vi "Stop Core.vi"(10 "final error code":i32, 11 "Acquisition in":refnum<class "Acquisition.lvclass">) -> (3 "Acquisition out":refnum<class "Acquisition.lvclass">)   [LabVIEW 2018, in "Acquisition.lvlib" / "Acquisition.lvclass"]
doc: "(<B>Filename</B>: Actor Framework.lvlib:Actor.lvclass:Stop Core.vi)\n\nDefines what the actor does before it stops. Use the <B>final error code</B> input to determine whether the actor shut down in response to an error.\n\nBy default, this method passes the Stop message along to all auto-stop nested actors. A descendant class may override this method to define additional behavior, such as shutting down any processes the actor initiated in its override of the Actor Core method."
uses:
  Acquisition.lvclass
  Acquisition.lvclass/Acquisition.ctl
  <vilib>/ActorFramework/Actor/Actor.lvclass
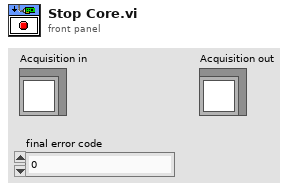
[diagram p1: front panel]
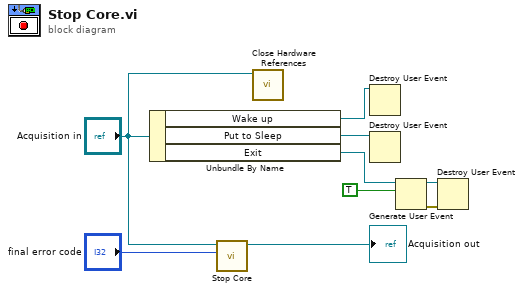
[diagram p0: block diagram]
diagram:
  n1 = Unbundle By Name("Acquisition in") -> ("Wake up"=w8:refnum<user-event>, "Put to Sleep"=w7:refnum<user-event>, "Exit"=w6:refnum<user-event>)
  n2 = call-parent "Stop Core.vi"("final error code"="final error code", "Actor in"="Acquisition in") -> ("Actor out"=→"Acquisition out":refnum<class "Acquisition.lvclass">)  [unwired: 9 in]
  n3 = call-dynamic "Close Hardware References.vi"("Acquisition in"="Acquisition in") -> ()  [unwired: 9 in, 2 out]
  n4 = Destroy User Event(user event=w8) -> ()  [unwired: 1 in, 1 out]
  n5 = Destroy User Event(user event=w7) -> ()  [unwired: 1 in, 1 out]
  n6 = Generate User Event(user event=w6, event data cluster=TRUE ("event data")) -> (user event out=w4:refnum<user-event>, error out=w3:errorcluster)  [unwired: 2 in]
  n7 = Destroy User Event(user event=w4, error in=w3) -> ()  [unwired: 1 out]
